vi "DropIn Show Button Help.vi"(0 "VI Refnum":refnum<vi>, 11 "error in (no error)":errorcluster) -> (15 "error out":errorcluster)   [LabVIEW 2011]
doc: "This is a demonstration of a very simple drop in that will call a message box which displays the control documentation when ever the user right clicks on a control.\n\nYou must terminate this drop in by pressing a boolean button labeled as \"Exit\" in the calling VI.\n\nAAL 9/09"
uses:
  <vilib>/Utility/traverseref.llb/TRef TravTarget.ctl
  <vilib>/Utility/traverseref.llb/VI Scripting - Traverse.lvlib
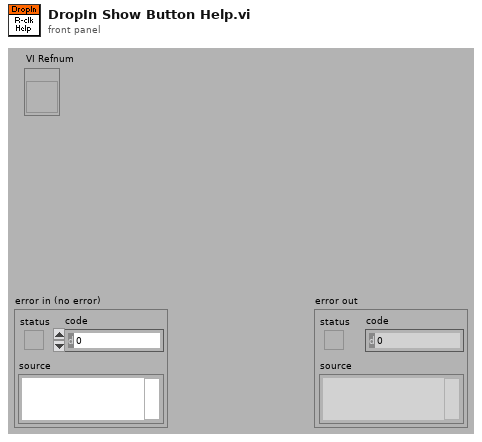
[diagram p1: front panel]
types:
  T1 = typedef "TRef TravTarget.ctl" = enum16{"FP", "BD", "Other"}
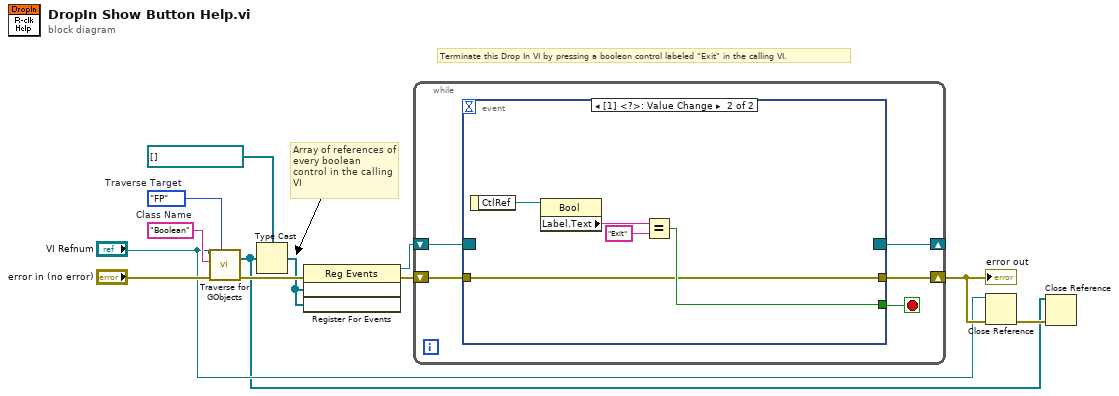
[diagram p0: block diagram]
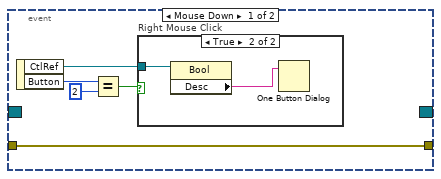
[diagram p2: hidden frame]
diagram:
  w12 = TRef_TravTarget."FP"  # Traverse Target
  w11 = "Boolean"  # Class Name
  # "Array of references of every boolean control in the calling VI"
  # "Terminate this Drop In VI by pressing a booleon control labeled \"Exit\" in the calling VI."
  n1 = call <vilib>:"Traverse for GObjects.vi"("Traverse Target"=w12, "error in (no error)"="error in (no error)", "Class Name"=w11, "VI Refnum"="VI Refnum") -> ("error out"=w7:errorcluster, "References"=w1:refnum<vi>[])  [unwired: 4 in, 2 out]
  n2 = Type Cast(type=refnum<vi>[] [], x=w1) -> (*(type *) &x=w3:refnum<vi>[])
  n3 = register-events(error in=w7, w3, w3) -> (reference out=w10:refnum<event-registration>, error out=w9:errorcluster)  [unwired: 1 in]
  n4 = while {
    shift-right: [w14] -> _
    shift-left: w10 -> [w17]
    shift-right: [w15] -> w6
    shift-left: w9 -> [w16]
    stop <- w13 stop-if-true
    n5 = event shown="[1] <?>: Value Change" {
      selector: w17 -> [_ _]
      dyn-events: [_ _] -> w14
      timeout: _ -> [_ _]
      tunnel: w16 -> [w18 w25]
      tunnel: [w18 w25] -> w15
      tunnel: [_ w26] -> w13
      event Mouse Down {
        n6 = event-data() -> ("CtlRef"=w22:refnum<vi>, "Button"=w21:u16)  [unwired: 1 out]
        n7 = Equal?(x=w21, y=u16 2) -> (x = y?=w19:bool)
        n8 = case "Right Mouse Click" shown="True" w19 {
          tunnel: w22 -> [_ w24]
          frame False {
          }
          frame True {
            n9 = property class="Bool"(reference=w24) -> ("Desc"=w23:string)  [unwired: 1 in, 2 out]
            n10 = One Button Dialog(message=w23) -> ()  [unwired: 2 out]
          }
        }
      }
      event Value Change {
        n11 = event-data() -> ("CtlRef"=w27:refnum<vi>)  [unwired: 1 out]
        n12 = property class="Bool"(reference=w27) -> ("Label.Text"=w29:string)  [unwired: 1 in, 2 out]
        n13 = Equal?(x=w29, y="Exit") -> (x = y?=w26:bool)
      }
    }
  }
  "error out" <- w6
  n14 = Close Reference(reference="VI Refnum", error in (no error)=w6) -> (error out=w2:errorcluster)
  n15 = Close Reference(reference=w1, error in (no error)=w2) -> ()  [unwired: 1 out]
